vi "HTTP add headers.vi"(11 "error in (no error)":errorcluster) -> (4 "client handle out":T1, 15 "error out":errorcluster)   [LabVIEW 2015, in "InfluxDB Client.lvclass"]
doc: "Adds HTTP headers for JSON content and encoding."
uses:
  InfluxDB Client.lvclass
  <vilib>/httpClient/ClientHandle.ctl
  <vilib>/httpClient/LabVIEWHTTPClient.lvlib
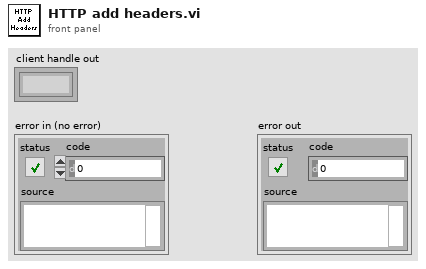
[diagram p1: front panel]
types:
  T1 = typedef "LabVIEWHTTPClient.lvlib/ClientHandle.ctl" = refnum<k1>
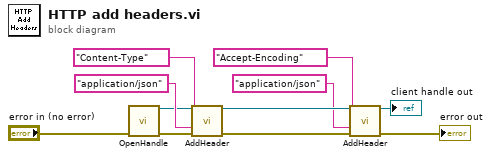
[diagram p0: block diagram]
diagram:
  n1 = call <vilib>:"OpenHandle.vi"("error in (no error)"="error in (no error)") -> ("client handle out"=w3:T1, "error out"=w4:errorcluster)  [unwired: 13 in]
  n2 = call <vilib>:"AddHeader.vi"("client handle"=w3, "header"="Content-Type", "value"="application/json", "error in (no error)"=w4) -> ("client handle out"=w9:T1, "error out"=w10:errorcluster)  [unwired: 10 in]
  n3 = call <vilib>:"AddHeader.vi"("client handle"=w9, "header"="Accept-Encoding", "value"="application/json", "error in (no error)"=w10) -> ("client handle out"=→"client handle out":T1, "error out"=→"error out":errorcluster)  [unwired: 10 in]
